vi "CameraCheckUpdate.vi"(8 "error constant":errorcluster) -> (0 "error constant 2":errorcluster)   [LabVIEW 2019]
uses:
  GlobalCamSettings.vi
  Global.lvlib
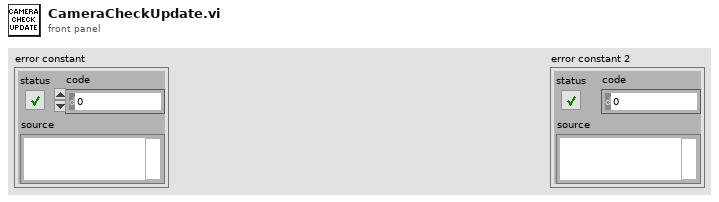
[diagram p1: front panel]
types:
  T1 = typedef "CameraSettings.ctl" = cluster{"EM Gain :":dbl, "Pre Amp Gain :":dbl, "VS Speed [Index] :":dbl, "VS Amplitude :":dbl, "Exposure Time [s] :":dbl, "Temperature :":dbl, "HS Speed [s]":dbl, "Gain > 300 :":bool}
  T2 = cluster{"EM Gain :":bool, "Pre Amp Gain :":bool, "VS Speed [Index] :":bool, "VS Amplitude :":bool, "Exposure Time [s] :":bool, "Temperature :":bool, "HS Speed [s]":bool, "Gain > 300 :":bool}
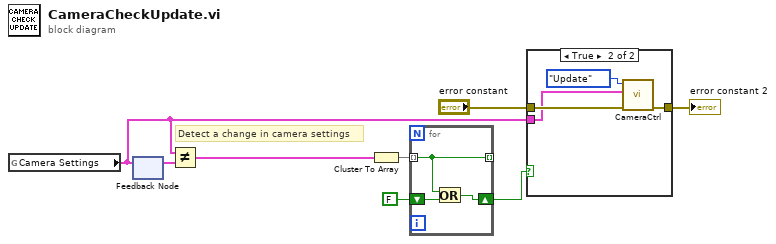
[diagram p0: block diagram]
diagram:
  # "Detect a change in camera settings"
  n1 = global read "GlobalCamSettings.vi" "Camera Settings"() -> (w1:T1)
  n2 = feedback #1() -> (w4:T1)  [unwired: 1 in]
  n3 = feedback-in #1(w1) -> ()
  n4 = Not Equal?(x=w1, y=w4) -> (x != y?=w5:T2)
  n5 = Cluster To Array(cluster=w5) -> (array=w6:bool[])
  n6 = for {
    tunnel: [w11] -> _ mode=indexing
    tunnel: w6 -> [w11] mode=indexing
    shift-right: [w9] -> w8
    shift-left: FALSE -> [w10]
    n7 = Or(x=w11, y=w10) -> (x .or. y?=w9:bool)
  }
  n8 = case shown="True" w8 {
    tunnel: "error constant" -> [w12 w15]
    tunnel: [w12 w14] -> w2
    tunnel: w1 -> [_ w13]
    frame False {
    }
    frame True {
      n9 = call "CameraCtrl.vi"("error constant"=w15, "Camera Settings"=w13, "Enum"=enum16{"Start", "Stop", "Acquire", "Update"}."Update") -> ("error constant 2"=w14:errorcluster)  [unwired: 6 in, 2 out]
    }
  }
  "error constant 2" <- w2
